vi "VsEP I-O Calibrator.vi"(11 "Data Folder":path=path "C:/Data/XYZ DATA/XYZ999") -> ()   [LabVIEW 2020]
uses:
  Typedefs/VsEP-Hidden Params.ctl
  epl-vi-lib/Signal Synthesis VIs/Controls/Gate XCtl/Gate Control.xctl
  Typedefs/VsEPCal- Stimulus.ctl
  Typedefs/VsEPCal-Parameters.ctl
panel:
  in  "Start Button":bool
  in  "Stop Button":bool
  in  "Adjust amp":bool
  in  "Response":T1={"Accelerometer Sensitivity (mV/g)"=98.0, "#Averages"=250, "Time Window (ms)"=20.0, "Gain"=100.0} {"Accelerometer Sensitivity (mV/g)" format="%_6g"}
  in  "Stimulus":T2={"Rep rate (Hz)"=20.0, "Start (dB atten)"=60.0, "Stop (dB atten)"=10.0, "Step (dB)"=10.0}
  out "Max Jerk (dB re 1g/ms)":dbl=-inf
  out "Abort":bool
  in  "finished":errorcluster
  in  "Params":T3={"Stimulus"={"Rep rate (Hz)"=14.0, "Start (dB atten)"=60.0, "Stop (dB atten)"=10.0, "Step (dB)"=10.0}, "Response"={"Accelerometer Sensitivity (mV/g)"=24.0, "#Averages"=128, "Time Window (ms)"=20.0, "Gain"=40.0}, "Hidden"={"AO Sampling Rate (Hz)"=100000.0, "AI Sampling Rate (Hz)"=100000.0, "Masker Timing"={"Active"=FALSE, "Delay (ms)"=0.0, "Width (ms)"=0.0, "Ramp (ms)"=0.0}, "Jerk rise time (ms)"=2.0, "Masker atten"=0.0, "show adjust"=FALSE, "linear gain"=FALSE}}
  out "mV from Accelerometer":dbl format="%#_4g"
  out "Attenuation (dB)":dbl format="%#_4g"
  out "Nonlinear":cluster{i32, dbl, dbl[][]}(graph)={0, 0.04, []}
  out "Linear":cluster{i32, dbl, dbl[][]}(graph)={0, 0.04, []}
  out "I-O graph":cluster{"array":ext[], "array":ext[]}[](graph)
  in  "Hidden":T4={"AO Sampling Rate (Hz)"=100000.0, "AI Sampling Rate (Hz)"=100000.0, "Masker Timing"={"Active"=FALSE, "Delay (ms)"=0.0, "Width (ms)"=0.0, "Ramp (ms)"=0.0}, "Jerk rise time (ms)"=2.0, "Masker atten"=0.0, "show adjust"=FALSE, "linear gain"=FALSE}
  # "Accelerometer Sensitivity\nKnowles use  24.0 mV/g\nEndevco Sensitivity 98.0  mV/g"
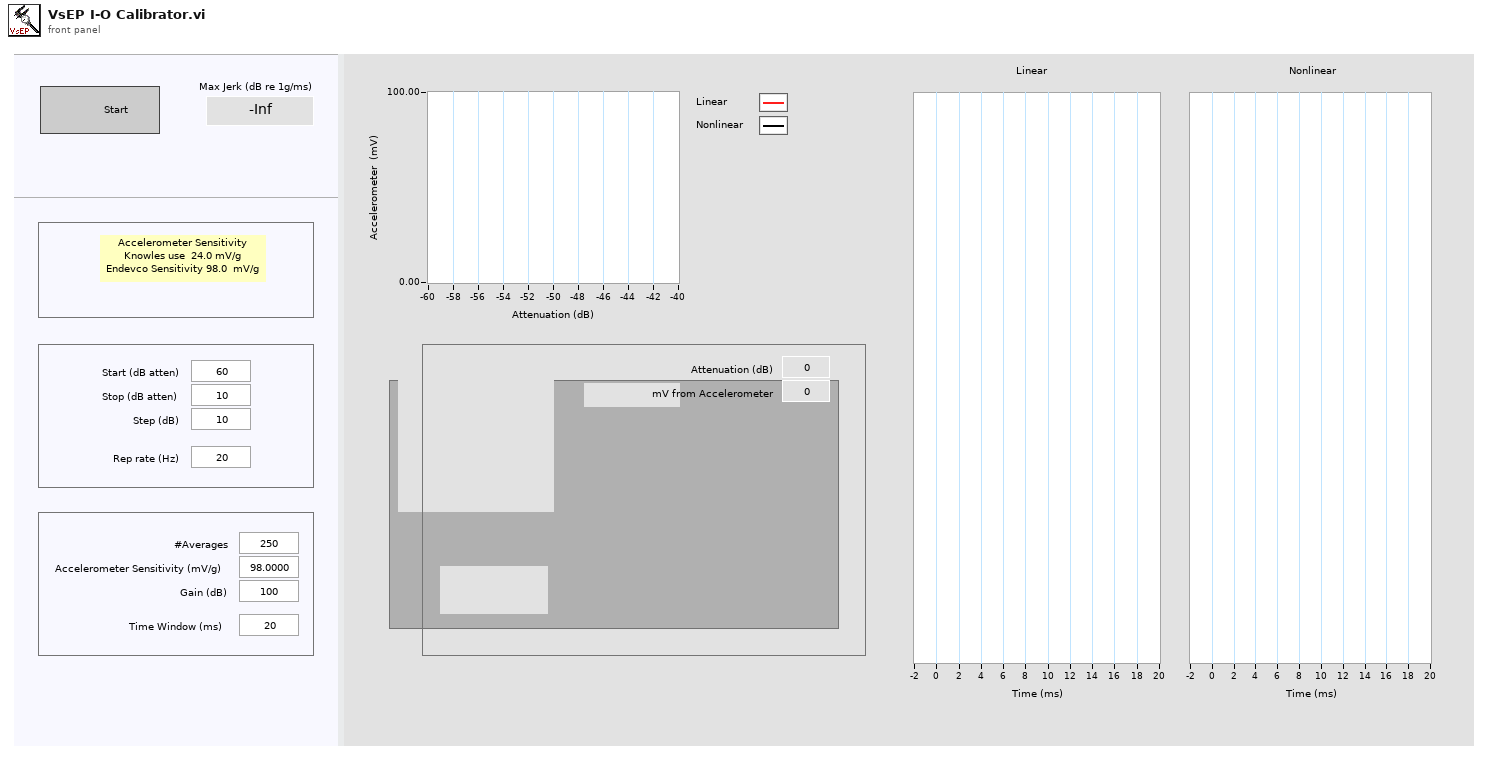
[diagram p1: front panel]
types:
  T1 = cluster{"Accelerometer Sensitivity (mV/g)":dbl, "#Averages":i32, "Time Window (ms)":dbl, "Gain":dbl}
  T2 = typedef "VsEPCal- Stimulus.ctl" = cluster{"Rep rate (Hz)":dbl, "Start (dB atten)":dbl, "Stop (dB atten)":dbl, "Step (dB)":dbl}
  T3 = typedef "VsEPCal-Parameters.ctl" = cluster{"Stimulus":T2, "Response":cluster{"Accelerometer Sensitivity (mV/g)":dbl, "#Averages":i32, "Time Window (ms)":dbl, "Gain":dbl}, "Hidden":T4}
  T4 = typedef "VsEP-Hidden Params.ctl" = cluster{"AO Sampling Rate (Hz)":dbl, "AI Sampling Rate (Hz)":dbl, "Masker Timing":cluster{"Active":bool, "Delay (ms)":dbl, "Width (ms)":dbl, "Ramp (ms)":dbl}, "Jerk rise time (ms)":dbl, "Masker atten":dbl, "show adjust":bool, "linear gain":bool}
  T5 = typedef "VsEP-Runtime Data.ctl" = cluster{"chan":i32[], "Ceiling":dbl, "dt (us)":dbl, "Crossed?":bool, "Step":dbl, "Stop":i32, "Avgs":i32, "Level":dbl, "AI Npts":i32, "Doubled?":bool, "reps/frame":i32, "altpol":bool, "AO npts":i32, "win Npts":i32, "gain":dbl}
  T6 = typedef "VsEP-Response Control.ctl" = cluster{"Grass Gain":i32, "#AVERAGES":i32, "Time Window (ms)":sgl, "Fast Steps Threshold":i32}
  T7 = cluster{"Stimulus":T2, "Response":cluster{"Accelerometer Sensitivity (mV/g)":dbl, "#Averages":i32, "Time Window (ms)":dbl, "Gain":dbl}, "Hidden":T4}
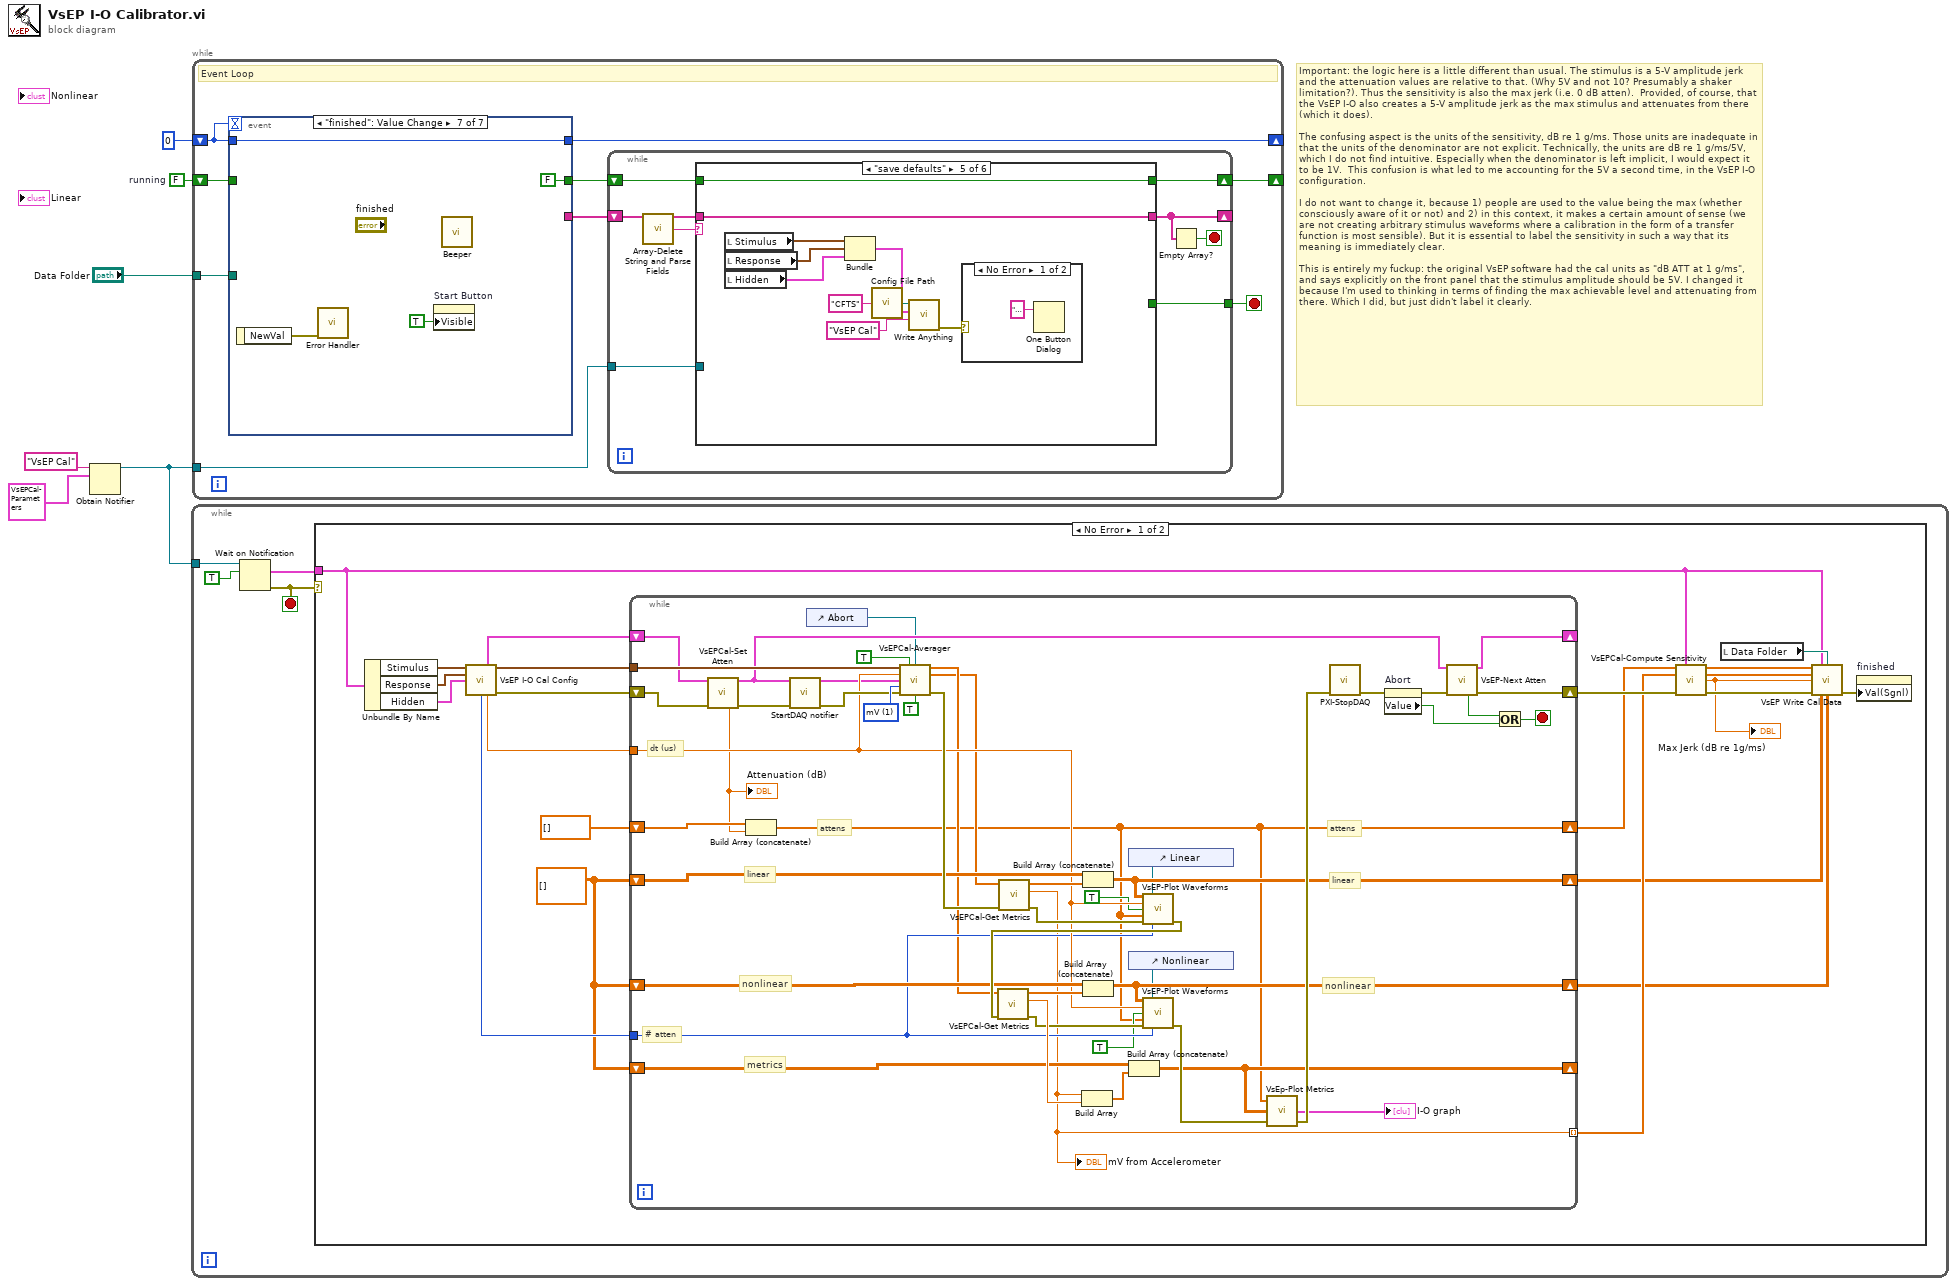
[diagram p0: block diagram]
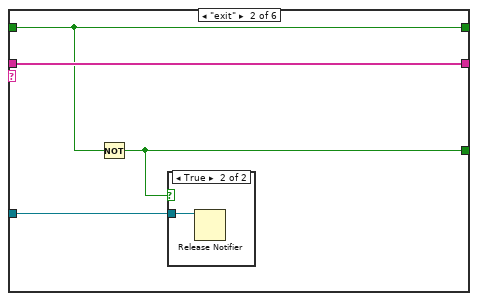
[diagram p4: hidden frame]
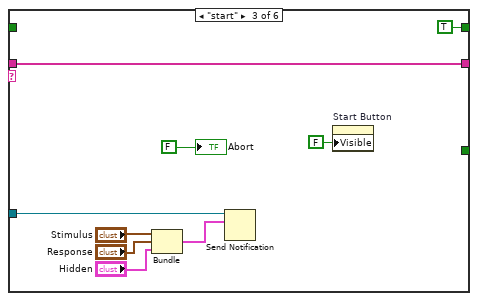
[diagram p6: hidden frame]
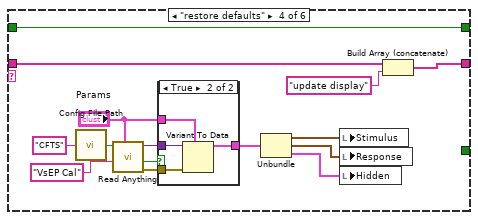
[diagram p7: hidden frame]
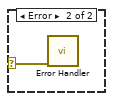
[diagram p9: hidden frame]
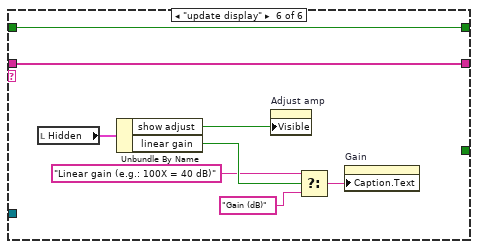
[diagram p10: hidden frame]
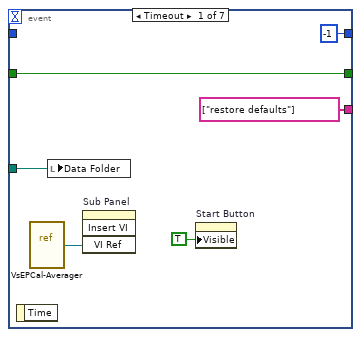
[diagram p11: hidden frame]
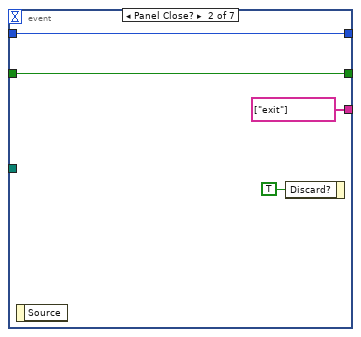
[diagram p12: hidden frame]
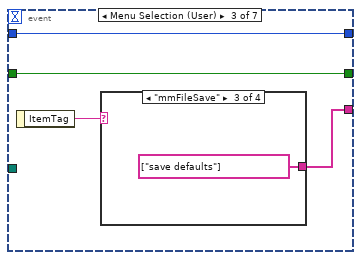
[diagram p13: hidden frame]
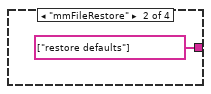
[diagram p15: hidden frame]
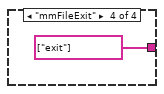
[diagram p16: hidden frame]
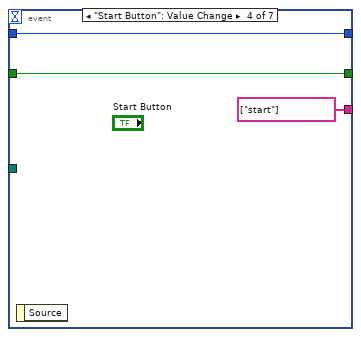
[diagram p17: hidden frame]
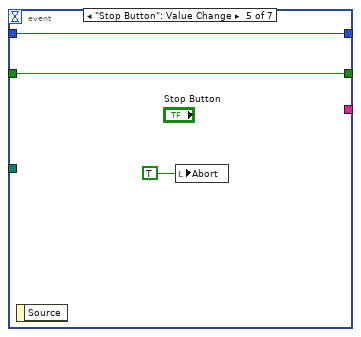
[diagram p18: hidden frame]
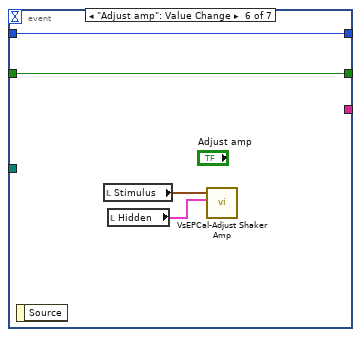
[diagram p19: hidden frame]
diagram:
  w1 = FALSE  # running
  # "Important: the logic here is a little different than usual. The stimulus is a 5-V amplitude jerk and the attenuation values are relative to that. (Why 5V and not 10? Presumably a shaker limitation?). Thus the sensitivity is also the max jerk (i.e. 0 dB atten).  Provided, of course, that the VsEP I-O also creates a 5-V amplitude jerk as the max stimulus and attenuates from there (which it does).\n\nThe confusing aspect is the units of the sensitivity, dB re 1 g/ms. Those units are inadequate in that the units of the denominator are not explicit. Technically, the units are dB re 1 g/ms/5V, which I do not find intuitive. Especially when the denominator is left implicit, I would expect it to be 1V.  This confusion is what led to me accounting for the 5V a second time, in the VsEP I-O configuration.\n\nI do not want to change it, because 1) people are used to the value being the max (whether consciously aware of it or not) and 2) in this context, it makes a certain amount of sense (we are not creating arbitrary stimulus waveforms where a calibration in the form of a transfer function is most sensible). But it is essential to label the sensitivity in such a way that its meaning is immediately clear.\n\nThis is entirely my fuckup: the original VsEP software had the cal units as \"dB ATT at 1 g/ms\", and says explicitly on the front panel that the stimulus amplitude should be 5V. I changed it because I'm used to thinking in terms of finding the max achievable level and attenuating from there. Which I did, but just didn't label it clearly."
  n1 = Obtain Notifier(name (unnamed)="VsEP Cal", notification data type=T3 {"Stimulus"={"Rep rate (Hz)"=0.0, "Start (dB atten)"=0.0, "Stop (dB atten)"=0.0, "Step (dB)"=0.0}, "Response"={"Accelerometer Sensitivity (mV/g)"=0.0, "#Averages"=0, "Time Window (ms)"=0.0, "Gain"=0.0}, "Hidden"={"AO Sampling Rate (Hz)"=0.0, "AI Sampling Rate (Hz)"=0.0, "Masker Timing"={"Active"=FALSE, "Delay (ms)"=0.0, "Width (ms)"=0.0, "Ramp (ms)"=0.0}, "Jerk rise time (ms)"=0.0, "Masker atten"=0.0, "show adjust"=FALSE, "linear gain"=FALSE}} ("Params")) -> (notifier out=w6:refnum<notifier>)  [unwired: 2 in, 2 out]
  n2 = while {
    tunnel: w6 -> [w9]
    stop <- w8 stop-if-true
    n3 = Wait on Notification(notifier=w9, ignore previous (F)=TRUE) -> (notification=w7:T3, error out=w8:errorcluster)  [unwired: 2 in, 2 out]
    n4 = case shown="No Error" w8 {
      tunnel: w7 -> [w15 _]
      frame No Error {
        w21 = dbl[][] []
        n5 = Unbundle By Name(w15) -> ("Stimulus"=w14:T2, "Response"=w13:T1, "Hidden"=w12:T4)
        n6 = call "VsEP I-O Cal Config.vi"("Stimulus"=w14, "Response"=w13, "Hidden"=w12) -> ("Runtime"=w28:T5, "RESPONSE"=w32:T6, "Num Atten"=w29:i32, "AI Sampling Interval (us)"=w30:dbl, "error out"=w31:errorcluster)  [unwired: 8 in]
        n7 = while {
          tunnel: w32 -> [w54]
          shift-right: [w62] -> w24
          shift-left: w21 -> [w64]
          shift-right: [w34] -> w25
          shift-left: dbl[] [] -> [w63]
          shift-right: [w60] -> w23
          shift-left: w21 -> [w61]
          shift-right: [w57] -> _
          shift-left: w21 -> [w58]
          tunnel: w30 -> [w53]
          tunnel: w29 -> [w52]
          shift-right: [w41] -> _
          shift-left: w28 -> [w51]
          tunnel: [w39] -> w26 mode=indexing
          shift-right: [w43] -> w27
          shift-left: w31 -> [w50]
          stop <- w46 stop-if-true
          w77 = 1 items=["Volts", "mV", "uV"] ("Output Scaling")
          # "# atten"
          # "dt (us)"
          # "attens"
          # "attens"
          # "nonlinear"
          # "linear"
          # "metrics"
          # "nonlinear"
          # "linear"
          n8 = call "VsEPCal-Set Atten.vi"("Runtime"=w51, "error in (no error)"=w50) -> ("Runtime out"=w40:T5, "Level"=w48:dbl, "error out"=w49:errorcluster)  [unwired: 11 in]
          "Attenuation (dB)" <- w48
          n9 = Build Array (concatenate)(w63, w48) -> (w34:dbl[])
          n10 = call "StartDAQ notifier.vi"("error in (no error)"=w49) -> ("error out"=w75:errorcluster)  [unwired: 6 in]
          n11 = control-ref of="Abort"() -> (w33:refnum<vi>)
          n12 = call "VsEPCal-Averager.vi"("Response"=w54, "flip polarity?"=TRUE, "Abort"=w33, "sample interval (us)"=w53, "Runtime"=w40, "Output Scaling"=w77, "error in (no error)"=w75, "Reject\nOverRide"=TRUE ("Reject\nOverRide")) -> ("Neural (uV)"=w38:dbl[], "microphonic (uV)"=w37:dbl[], "error out"=w66:errorcluster)  [unwired: 3 in, 2 out]
          n13 = call "VsEPCal-Get Metrics.vi"("error in (no error)"=w66, "Data in"=w37) -> ("error out"=w70:errorcluster, "accelerometer (mV)"=w39:dbl, "Data out"=w71:dbl[])  [unwired: 7 in]
          "mV from Accelerometer" <- w39
          n14 = Build Array (concatenate)(w64, w71) -> (w62:dbl[][])
          n15 = control-ref of="Linear"() -> (w56:refnum<vi>)
          n16 = control-ref of="Nonlinear"() -> (w55:refnum<vi>)
          n17 = call "VsEP-Plot Waveforms.vi"("Array"=w62, "graph ref"=w56, "dt (us)"=w53, "Normalize traces"=TRUE, "Sequence values"=w34, "error in (no error)"=w70, "Max #SPL"=w52) -> ("error out"=w69:errorcluster)  [unwired: 7 in, 1 out]
          n18 = call "VsEPCal-Get Metrics.vi"("error in (no error)"=w69, "Data in"=w38) -> ("error out"=w68:errorcluster, "accelerometer (mV)"=w74:dbl, "Data out"=w72:dbl[])  [unwired: 7 in]
          n19 = Build Array(w39, w74) -> (w67:dbl[])
          n20 = Build Array (concatenate)(w61, w72) -> (w60:dbl[][])
          n21 = Build Array (concatenate)(w58, w67) -> (w57:dbl[][])
          n22 = call "VsEP-Plot Waveforms.vi"("Array"=w60, "graph ref"=w55, "dt (us)"=w53, "Normalize traces"=TRUE, "Sequence values"=w34, "error in (no error)"=w68, "Max #SPL"=w52) -> ("error out"=w73:errorcluster)  [unwired: 7 in, 1 out]
          n23 = call "VsEp-Plot Metrics.vi"("error in (no error)"=w73, "metrics"=w57, "level"=w34) -> ("error out"=w65:errorcluster, "appended array"=→"I-O graph":cluster{"array":ext[], "array":ext[]}[])  [unwired: 1 in]
          n24 = call "PXI-StopDAQ.vi"("error in (no error)"=w65) -> ("error out"=w45:errorcluster)  [unwired: 6 in]
          n25 = property on="Abort" class="Bool (strict)"(error in=w45) -> (error out=w44:errorcluster, "Value"=w47:bool)  [unwired: 1 in, 1 out]
          n26 = call "VsEP-Next Atten.vi"("Runtime"=w40, "error in (no error)"=w44) -> ("Runtime out"=w41:T5, "Finished"=w42:bool, "error out"=w43:errorcluster)  [unwired: 11 in]
          n27 = Or(x=w42, y=w47) -> (x .or. y?=w46:bool)
        }
        n28 = call "VsEPCal-Compute Sensitivity.vi"("Atten (dB)"=w25, "Params"=w15, "accelerometer (mV)"=w26, "error in (no error)"=w27) -> ("Atten (dB) thru"=w18:dbl[], "accelerometer (mV) thru"=w17:dbl[], "Max Jerk (dB re 1g/ms)"=w19:dbl, "error out"=w20:errorcluster)  [unwired: 8 in]
        "Max Jerk (dB re 1g/ms)" <- w19
        n29 = local read "Data Folder"() -> (w16:path)
        n30 = call "VsEP Write Cal Data.vi"("Atten (dB)"=w18, "Params"=w15, "Data Folder"=w16, "accelerometer (mV)"=w17, "Sensitivity"=w19, "error in (no error)"=w20, "Linear"=w24, "Nonlinear"=w23) -> ("error out"=w11:errorcluster)  [unwired: 7 in]
        n31 = property on="finished" class="Clust (strict)"("Val(Sgnl)"=w11) -> ()  [unwired: 2 in, 2 out]
      }
      frame Error {
      }
    }
  }
  n32 = while {
    tunnel: w6 -> [w84]
    shift-right: [w87] -> _
    shift-left: 0 -> [w85]
    tunnel: "Data Folder" -> [w86]
    shift-right: [w81] -> _
    shift-left: w1 -> [w79]
    stop <- w82 stop-if-true
    # "Event Loop"
    n33 = event shown="[6] \"finished\": Value Change" {
      selector: _ -> [_ _ _ _ _ _ _]
      dyn-events: _ -> [_ _ _ _ _ _ _]
      timeout: w85 -> [_ _ _ _ _ _ _]
      tunnel: [-1 w162 w166 w172 w174 w177 w183] -> w87
      tunnel: w86 -> [w156 _ _ _ _ _ _]
      tunnel: w85 -> [_ w162 w166 w172 w174 w177 w183]
      tunnel: [string[] ["restore defaults"] string[] ["exit"] w163 string[] ["start"] _ _ _] -> w83
      tunnel: [w153 w160 w164 w170 w173 w176 FALSE ("running")] -> w80
      tunnel: w79 -> [w153 w160 w164 w170 w173 w176 _]
      event Timeout {
        n34 = event-data() -> ()  [unwired: 1 in, 1 out]
        n35 = vi-ref "VsEPCal-Averager.vi"() -> (w158:refnum<vi>)
        n36 = local write "Data Folder"(w156) -> ()
        n37 = invoke on="Sub Panel" class="SubPanel" method="Insert VI"("VI Ref"=w158) -> ()  [unwired: 3 in, 4 out]
        n38 = property on="Start Button" class="Bool"("Visible"=TRUE) -> ()  [unwired: 2 in, 2 out]
      }
      event Panel Close? {
        n39 = event-data() -> ()  [unwired: 1 in, 1 out]
        n40 = event-data("Discard?"=TRUE) -> ()  [unwired: 1 in, 1 out]
      }
      event Menu Selection (User) {
        n41 = event-data() -> ("ItemTag"=w165:string)  [unwired: 1 in]
        n42 = case shown="\"mmFileSave\"" w165 {
          tunnel: [_ string[] ["restore defaults"] string[] ["save defaults"] string[] ["exit"]] -> w163
          frame "", Default {
          }
          frame "mmFileRestore" {
          }
          frame "mmFileSave" {
          }
          frame "mmFileExit" {
          }
        }
      }
      event "Start Button": Value Change {
        n43 = event-data() -> ()  [unwired: 1 in, 1 out]
      }
      event "Stop Button": Value Change {
        n44 = event-data() -> ()  [unwired: 1 in, 1 out]
        n45 = local write "Abort"(TRUE ("Stopping")) -> ()
      }
      event "Adjust amp": Value Change {
        n46 = event-data() -> ()  [unwired: 1 in, 1 out]
        n47 = local read "Stimulus"() -> (w179:T2)
        n48 = local read "Hidden"() -> (w178:T4)
        n49 = call "VsEPCal-Adjust Shaker Amp.vi"("Hidden"=w178, "Stimulus"=w179) -> ()  [unwired: 10 in]
      }
      event "finished": Value Change {
        n50 = event-data() -> ("NewVal"=w182:errorcluster)  [unwired: 1 in]
        n51 = call "Error Handler.vi"("error in (no error)"=w182) -> ()  [unwired: 13 in, 2 out]
        n52 = property on="Start Button" class="Bool"("Visible"=TRUE) -> ()  [unwired: 2 in, 2 out]
        n53 = call "Beeper.vi"() -> ()  [unwired: 5 in, 1 out]
      }
    }
    n54 = while {
      shift-right: [w96] -> _
      shift-left: w83 -> [w93]
      tunnel: [w94] -> w82
      tunnel: w84 -> [w90]
      shift-right: [w89] -> w81
      shift-left: w80 -> [w88]
      stop <- w95 stop-if-true
      n55 = call "Array-Delete String and Parse Fields.vi"("Array in"=w93) -> ("Array out"=w92:string[], "Field 1"=w91:string)  [unwired: 10 in, 3 out]
      n56 = case shown="\"save defaults\"" w91 {
        tunnel: w92 -> [w98 w102 w112 w127 w142 w152]
        tunnel: [w98 w102 w112 w114 w142 w152] -> w96
        tunnel: [_ w99 _ _ _ _] -> w94
        tunnel: w90 -> [_ w101 w108 _ _ _]
        tunnel: [w97 w100 TRUE ("running") w117 w138 w151] -> w89
        tunnel: w88 -> [w97 w100 _ w117 w138 w151]
        frame "", Default {
        }
        frame "exit" {
          n57 = Not(x=w100) -> (.not. x?=w99:bool)
          n58 = case shown="True" w99 {
            tunnel: w101 -> [_ w103]
            frame False {
            }
            frame True {
              n59 = Release Notifier(notifier=w103) -> ()  [unwired: 2 in, 3 out]
            }
          }
        }
        frame "start" {
          n60 = Bundle("Stimulus"="Stimulus", "Response"="Response", "Hidden"="Hidden") -> (w107:T7)  [unwired: 1 in]
          n61 = Send Notification(notification=w107, notifier=w108) -> ()  [unwired: 1 in, 2 out]
          n62 = property on="Start Button" class="Bool"("Visible"=FALSE) -> ()  [unwired: 2 in, 2 out]
          "Abort" <- FALSE ("quitting")
        }
        frame "restore defaults" {
          n63 = call "Config File Path.vi"("AppName"="CFTS") -> ("Default config file name"=w125:path)
          n64 = call "Read Anything.vi"("Type of Anything"="Params", "Section Name (Name of \"Type of Anything\")"="VsEP Cal" ("Section Name (Name of \"Type of Anything\")"), "Path (dialog)"=w125) -> ("Error Out"=w121:errorcluster, "Found?"=w123:bool, "Anything"=w122:variant)  [unwired: 6 in]
          n65 = case shown="True" w123 {
            tunnel: w122 -> [_ w132]
            tunnel: "Params" -> [w128 w130]
            tunnel: w121 -> [_ w131]
            tunnel: [w128 w129] -> w120
            frame False {
            }
            frame True {
              n66 = Variant To Data(error in=w131, type=w130, Variant=w132) -> (data=w129:T3)  [unwired: 1 out]
            }
          }
          n67 = Unbundle(w120) -> ("Stimulus"=w119:T2, "Response"=w118:T1, "Hidden"=w115:T4)
          n68 = local write "Stimulus"(w119) -> ()
          n69 = local write "Response"(w118) -> ()
          n70 = local write "Hidden"(w115) -> ()
          n71 = Build Array (concatenate)(w127, "update display") -> (w114:string[])
        }
        frame "save defaults" {
          n72 = local read "Stimulus"() -> (w137:T2)
          n73 = local read "Response"() -> (w136:T1)
          n74 = local read "Hidden"() -> (w135:T4)
          n75 = Bundle("Stimulus"=w137, "Response"=w136, "Hidden"=w135) -> (w134:T7)  [unwired: 1 in]
          n76 = call "Config File Path.vi"("AppName"="CFTS") -> ("Default config file name"=w140:path)
          n77 = call "Write Anything.vi"("Section Name (Name of \"Anything\")"="VsEP Cal" ("Section Name (Name of \"Type of Anything\")"), "Anything"=w134, "Path (dialog)"=w140) -> ("Error Out"=w133:errorcluster)  [unwired: 7 in, 1 out]
          n78 = case shown="No Error" w133 {
            selector: w133 -> [_ w144]
            frame No Error {
              n79 = One Button Dialog(message="Defaults saved.") -> ()  [unwired: 1 in, 1 out]
            }
            frame Error {
              n80 = call "Error Handler.vi"("error in (no error)"=w144) -> ()  [unwired: 13 in, 2 out]
            }
          }
        }
        frame "update display" {
          n81 = local read "Hidden"() -> (w150:T4)
          n82 = Unbundle By Name(w150) -> ("show adjust"=w149:bool, "linear gain"=w148:bool)
          n83 = property on="Adjust amp" class="Bool"("Visible"=w149) -> ()  [unwired: 2 in, 2 out]
          n84 = Select(t="Linear gain (e.g.: 100X = 40 dB)", s=w148, f="Gain (dB)") -> (s? t:f=w146:string)
          n85 = property on="Gain" class="DigNum (strict)"("Caption.Text"=w146) -> ()  [unwired: 2 in, 2 out]
        }
      }
      n86 = Empty Array?(array=w96) -> (empty?=w95:bool)
    }
  }
